vi "TCP Daemon.vi"(8 "UUID":string, 9 "data model":refnum<class "Device Data Model.lvclass">, 10 "transmission data unit":refnum<class "Transmission Data Unit.lvclass">, 11 "TCP slave in":refnum<class "TCP Slave.lvclass">) -> ()   [LabVIEW 2015, in "SubVIs.lvlib" / "TCP Slave.lvclass"]
doc: "This daemon waits for new connections and launches connection handlers as needed. It also obtains a local reference to the quit notification, and waits for that to occur."
uses:
  <vilib>/Modbus/subvis/Protocol/TCP/TCP Slave/TCP Slave.lvclass
  <vilib>/Modbus/subvis/Transmission Data Unit (ADU)/Transmission Data Unit/Transmission Data Unit.lvclass
  <vilib>/Modbus/subvis/Data and Functions/Device Data Model/Device Data Model.lvclass
  <vilib>/Modbus/subvis/Protocol/Interfaces/Network Slave/Network Slave.lvclass/Network Slave.ctl
  <vilib>/Modbus/subvis/Protocol/TCP/TCP Slave/TCP Slave.lvclass/TCP Slave.ctl
  <vilib>/Modbus/subvis/Protocol/TCP/TCP Slave/Remove Unused Connections.vi
  <vilib>/Modbus/subvis/Protocol/Interfaces/Network Slave/Network Slave.lvclass
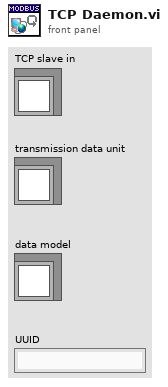
[diagram p1: front panel]
types:
  T1 = enum16{"Check Notifier", "Check for Available Connection Slot", "Wait on Connection", "Quit"}
  T2 = enum16{"Not Started", "Running", "Error", "Stopped"}
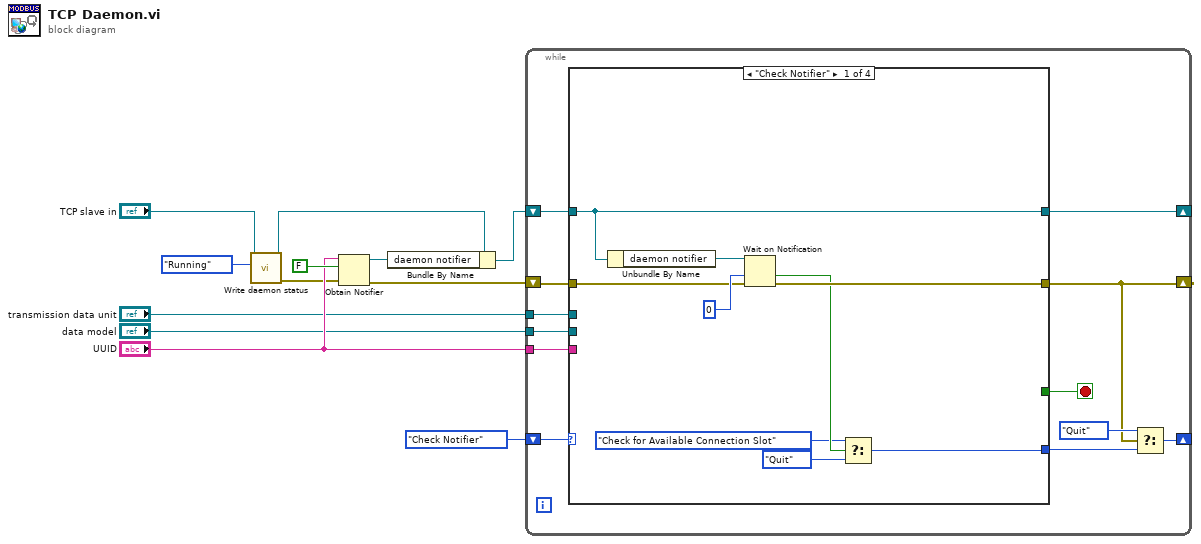
[diagram p0: block diagram]
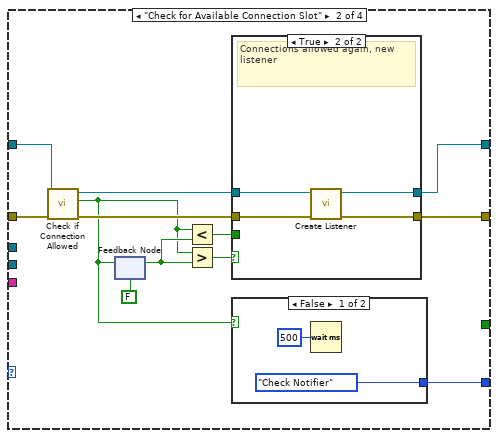
[diagram p2: hidden frame]
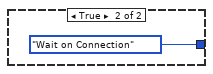
[diagram p3: hidden frame]
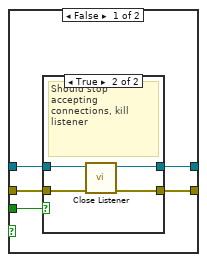
[diagram p4: hidden frame]
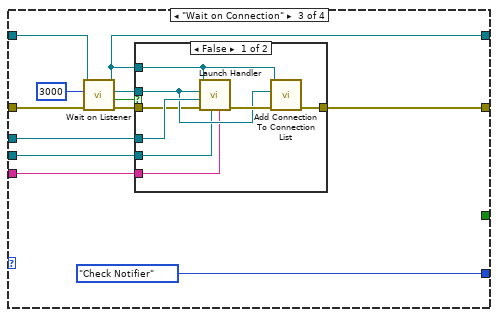
[diagram p6: hidden frame]
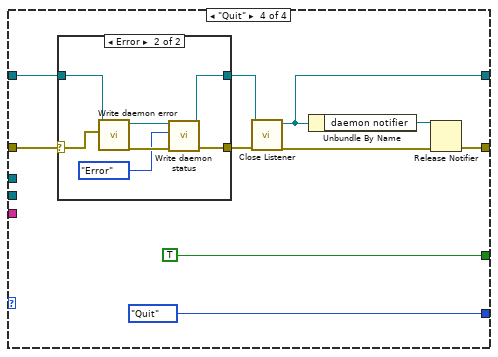
[diagram p8: hidden frame]
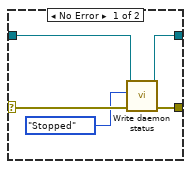
[diagram p9: hidden frame]
diagram:
  n1 = call <vilib>:"Write daemon status.vi"("daemon status"=T2."Running", "network slave in"="TCP slave in") -> ("error out"=w2:errorcluster, "network slave out"=w4:refnum<class "TCP Slave.lvclass">)  [unwired: 8 in]
  n2 = Obtain Notifier(name (unnamed)="UUID", notification data type=FALSE, error in (no error)=w2) -> (notifier out=w10:refnum<notifier>, error out=w5:errorcluster)  [unwired: 1 in, 1 out]
  n3 = Bundle By Name(cluster=w4, "daemon notifier"=w10) -> (w9:refnum<class "TCP Slave.lvclass">)
  n4 = while {
    shift-right: [w22] -> _
    shift-left: T1."Check Notifier" -> [w24]
    tunnel: "UUID" -> [w19]
    tunnel: "data model" -> [w18]
    tunnel: "transmission data unit" -> [w17]
    shift-right: [w16] -> _
    shift-left: w5 -> [w15]
    shift-right: [w13] -> _
    shift-left: w9 -> [w23]
    stop <- w14 stop-if-true
    n5 = case shown="\"Check Notifier\"" w24 {
      tunnel: w23 -> [w25 w44 w74 w93]
      tunnel: [w32 w38 w64 w90] -> w16
      tunnel: [w27 w34 T1."Check Notifier" T1."Quit"] -> w20
      tunnel: w19 -> [_ _ w71 _]
      tunnel: w18 -> [_ _ w70 _]
      tunnel: w17 -> [_ _ w69 _]
      tunnel: w15 -> [w26 w45 w68 w94]
      tunnel: [_ _ _ TRUE] -> w14
      tunnel: [w25 w39 w67 w85] -> w13
      frame "Check Notifier" {
        n6 = Unbundle By Name(w25) -> ("daemon notifier"=w33:refnum<notifier>)
        n7 = Wait on Notification(notifier=w33, timeout in ms (-1)=0, error in (no error)=w26) -> (timed out?=w31:bool, error out=w32:errorcluster)  [unwired: 1 in, 2 out]
        n8 = Select(t=T1."Check for Available Connection Slot", s=w31, f=T1."Quit") -> (s? t:f=w27:T1)
      }
      frame "Check for Available Connection Slot" {
        n9 = call <vilib>:"Check if Connection Allowed.vi"("error in (no error)"=w45, "TCP slave in"=w44) -> ("error out"=w41:errorcluster, "connection allowed"=w35:bool, "TCP slave out"=w40:refnum<class "TCP Slave.lvclass">)  [unwired: 7 in]
        n10 = feedback-in #1(w35) -> ()
        n11 = feedback #1(FALSE) -> (w37:bool)
        n12 = Less?(x=w35, y=w37) -> (x < y?=w36:bool)
        n13 = Greater?(x=w35, y=w37) -> (0:w42:bool)
        n14 = case shown="True" w42 {
          tunnel: w41 -> [w51 w62]
          tunnel: w40 -> [w52 w63]
          tunnel: [w49 w61] -> w39
          tunnel: [w50 w60] -> w38
          tunnel: w36 -> [w53 _]
          frame False {
            n15 = case shown="True" w53 {
              tunnel: w52 -> [w55 w59]
              tunnel: w51 -> [w54 w58]
              tunnel: [w54 w57] -> w50
              tunnel: [w55 w56] -> w49
              frame False {
              }
              frame True {
                # "Should stop accepting connections, kill listener"
                n16 = call <vilib>:"Close Listener.vi"("error in (no error)"=w58, "TCP slave in"=w59) -> ("error out"=w57:errorcluster, "TCP slave out"=w56:refnum<class "TCP Slave.lvclass">)  [unwired: 8 in]
              }
            }
          }
          frame True {
            # "Connections allowed again, new listener"
            n17 = call <vilib>:"Create Listener.vi"("error in (no error)"=w62, "TCP slave in"=w63) -> ("error out"=w60:errorcluster, "TCP slave out"=w61:refnum<class "TCP Slave.lvclass">)  [unwired: 8 in]
          }
        }
        n18 = case shown="False" w35 {
          tunnel: [T1."Check Notifier" T1."Wait on Connection"] -> w34
          frame False {
            n19 = Wait (ms)(milliseconds to wait=u32 500) -> ()  [unwired: 1 out]
          }
          frame True {
          }
        }
      }
      frame "Wait on Connection" {
        n20 = call-dynamic "Wait on Listener.vi"("error in (no error)"=w68, "timeout ms (wait forever: -1)"=3000, "TCP slave in"=w74) -> ("error out"=w65:errorcluster, "timed out?"=w66:bool, "connection reference"=w72:refnum<data-value>, "TCP slave out"=w67:refnum<class "TCP Slave.lvclass">)  [unwired: 5 in]
        n21 = case shown="False" w66 {
          tunnel: w72 -> [w80 _]
          tunnel: w67 -> [w79 _]
          tunnel: w71 -> [w78 _]
          tunnel: w70 -> [w77 _]
          tunnel: w69 -> [w83 _]
          tunnel: [w82 w84] -> w64
          tunnel: w65 -> [w76 w84]
          frame False {
            n22 = call <vilib>:"Launch Handler.vi"("UUID"=w78, "data model"=w77, "error in (no error)"=w76, "transmission data unit"=w83, "connection reference"=w80, "TCP slave"=w79) -> ("error out"=w81:errorcluster)  [unwired: 5 in]
            n23 = call <vilib>:"Add Connection To Connection List.vi"("error in (no error)"=w81, "data value reference"=w80, "TCP slave in"=w79) -> ("error out"=w82:errorcluster)  [unwired: 8 in]
          }
          frame True {
          }
        }
      }
      frame "Quit" {
        n24 = case shown="Error" w94 {
          selector: w94 -> [w96 w101]
          tunnel: [w97 w103] -> w92
          tunnel: w93 -> [w99 w106]
          tunnel: [w98 w104] -> w91
          frame No Error {
            n25 = call <vilib>:"Write daemon status.vi"("error in (no error)"=w96, "daemon status"=T2."Stopped", "network slave in"=w99) -> ("error out"=w97:errorcluster, "network slave out"=w98:refnum<class "TCP Slave.lvclass">)  [unwired: 7 in]
          }
          frame Error {
            n26 = call <vilib>:"Write daemon error.vi"("daemon error"=w101, "network slave in"=w106) -> ("error out"=w102:errorcluster, "network slave out"=w105:refnum<class "TCP Slave.lvclass">)  [unwired: 8 in]
            n27 = call <vilib>:"Write daemon status.vi"("error in (no error)"=w102, "daemon status"=T2."Error", "network slave in"=w105) -> ("error out"=w103:errorcluster, "network slave out"=w104:refnum<class "TCP Slave.lvclass">)  [unwired: 7 in]
          }
        }
        n28 = call <vilib>:"Close Listener.vi"("error in (no error)"=w92, "TCP slave in"=w91) -> ("error out"=w86:errorcluster, "TCP slave out"=w85:refnum<class "TCP Slave.lvclass">)  [unwired: 8 in]
        n29 = Unbundle By Name(w85) -> ("daemon notifier"=w87:refnum<notifier>)
        n30 = Release Notifier(notifier=w87, error in (no error)=w86) -> (error out=w90:errorcluster)  [unwired: 1 in, 2 out]
      }
    }
    n31 = Select(t=T1."Quit", s=w16, f=w20) -> (s? t:f=w22:T1)
  }
